vi "Grave Left Cell String.vi"(8 "Error In":errorcluster, 10 "Bookmark ID":u32, 11 "VI Path":path) -> (0 "Error Out":errorcluster, 1 "Bold?":bool, 2 "Color":u32(colorbox)=40705, 3 "Text":string)   [LabVIEW 2017, in "Bookmark Manager.lvlib"]
doc: "Gets the state name of the grave. If the Spirit frame is enabled, then the name is \"Spirit\". If the Corpse frame is enabled, then the name is \"Zombie\".\n\nThe Diagram Disable Structure cannot be obtained its label. The owning object of the label is the block diagram, not the Diagram Disable Structure that is attached to it. This means that all of the Diagram Disable structures in a VI must be searched by their label's UIDs to find the Diagram Disable Structure and determine its state."
uses:
  Bookmark Manager.lvlib
  <vilib>/Utility/traverseref.llb/TRef TravTarget.ctl
  Toolkit VIs/Public/Typedefs/Grave States.ctl
  <vilib>/Utility/traverseref.llb/VI Scripting - Traverse.lvlib
  Toolkit VIs/Toolkit VIs.lvlib
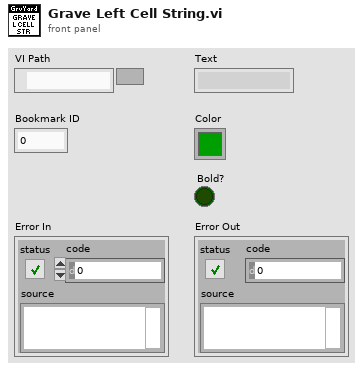
[diagram p1: front panel]
types:
  T1 = typedef "TRef TravTarget.ctl" = enum16{"FP", "BD", "Other"}
  T2 = typedef "Toolkit VIs.lvlib/Grave States.ctl" = enum16{"Spirit", "Zombie"}
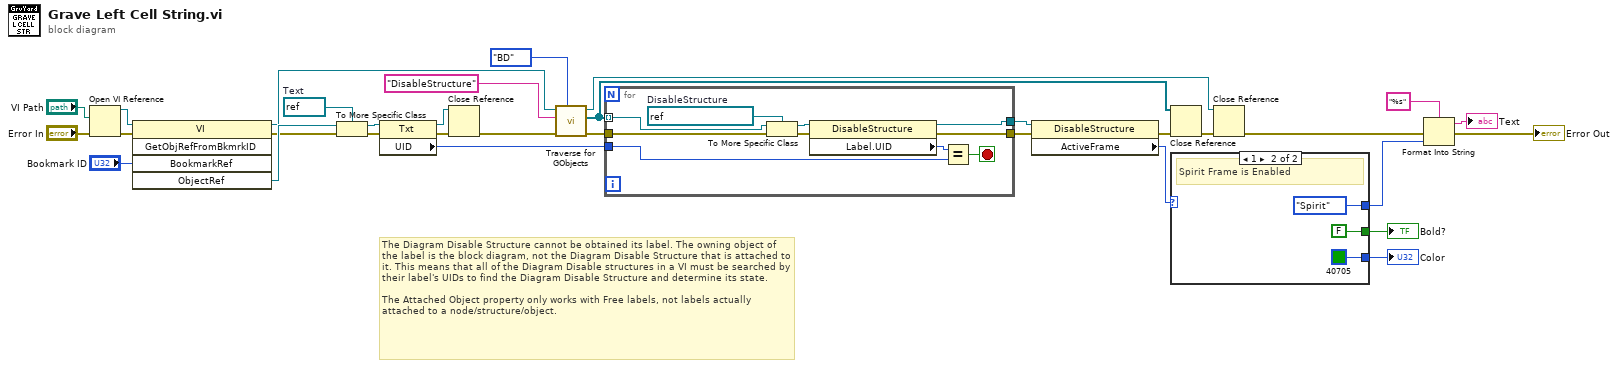
[diagram p0: block diagram]
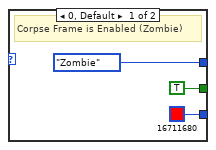
[diagram p2: hidden frame]
diagram:
  w21 = refnum<vi> refnum  # Text
  # "The Diagram Disable Structure cannot be obtained its label. The owning object of the label is the block diagram, not the Diagram Disable Structure that is attached to it. This means that all of the Diagram Disable structures in a VI must be searched by their label's UIDs to find the Diagram Disable Structure and determine its state.\n\nThe Attached Object property only works with Free labels, not labels actually attached to a node/structure/object."
  n1 = Open VI Reference(vi path="VI Path", error in (no error)="Error In") -> (vi reference=w13:refnum<vi>, error out=w14:errorcluster)  [unwired: 4 in]
  n2 = invoke class="VI" method="GetObjRefFromBkmrkID"(reference=w13, error in=w14, "BookmarkRef"="Bookmark ID") -> (reference out=w9:refnum<vi>, error out=w20:errorcluster, "ObjectRef"=w23:refnum<vi>)  [unwired: 2 in, 2 out]
  n3 = To More Specific Class(target class=w21, reference=w23, error in=w20) -> (specific class reference=w24:refnum<vi>, error out=w22:errorcluster)
  n4 = property class="Txt"(reference=w24, error in=w22) -> (reference out=w7:refnum<vi>, error out=w11:errorcluster, "UID"=w27:i32)
  n5 = Close Reference(reference=w7, error in (no error)=w11) -> (error out=w8:errorcluster)
  n6 = call <vilib>:"Traverse for GObjects.vi"("Traverse Target"=TRef_TravTarget."BD", "error in (no error)"=w8, "Class Name"="DisableStructure", "VI Refnum"=w9) -> ("error out"=w10:errorcluster, "References"=w32:refnum<vi>[], "dup VI Refnum"=w12:refnum<vi>)  [unwired: 4 in, 1 out]
  n7 = for {
    tunnel: w32 -> [w42] mode=indexing
    tunnel: w27 -> [w35]
    tunnel: w10 -> [w40]
    tunnel: [w38] -> w28
    tunnel: [w34] -> w30
    stop <- w33 stop-if-true
    w41 = refnum<vi> refnum  # DisableStructure
    n8 = To More Specific Class(target class=w41, reference=w42, error in=w40) -> (specific class reference=w37:refnum<vi>, error out=w39:errorcluster)
    n9 = property class="DisableStructure"(reference=w37, error in=w39) -> (reference out=w34:refnum<vi>, error out=w38:errorcluster, "Label.UID"=w36:i32)
    n10 = Equal?(x=w36, y=w35) -> (x = y?=w33:bool)
  }
  n11 = property class="DisableStructure"(reference=w30, error in=w28) -> (error out=w29:errorcluster, "ActiveFrame"=w31:i16)  [unwired: 1 out]
  n12 = Close Reference(reference=w32, error in (no error)=w29) -> (error out=w18:errorcluster)
  n13 = case shown="1" w31 {
    tunnel: [Grave_States."Zombie" ("Grave States") Grave_States."Spirit" ("Grave States")] -> w5
    tunnel: [u32 16711680 u32 40705] -> w1
    tunnel: [TRUE FALSE] -> w2
    frame 0, Default {
      # "Corpse Frame is Enabled (Zombie)"
    }
    frame 1 {
      # "Spirit Frame is Enabled"
    }
  }
  "Bold?" <- w2
  "Color" <- w1
  n14 = Close Reference(reference=w12, error in (no error)=w18) -> (error out=w19:errorcluster)
  n15 = Format Into String(format string="%s", error in=w19, w5) -> (resulting string=→"Text":string, error out=→"Error Out":errorcluster)  [unwired: 1 in]
